vi "CommonVIs_OneButtonDialog.vi"(1 "message":string, 3 "yesButtonName":string="OK", 4 "noButtonName":string="Cancel", 5 "error in (no error)":errorcluster, 6 "WindowTitle":string, 7 "timeout(-1 ms) -1=infinity":i32=-1) -> (13 "timeOut":bool=TRUE, 16 "yesButtonPressed":bool, 19 "error out":errorcluster)   [LabVIEW 2014]
doc: "Displays a dialog box that contains a message and two buttons. <B>yesButtonName</B> and <B>noButtonName</B> are the names displayed on the buttons of the dialog box."
panel:
  in  "yesButton":bool
  out "showMessage":string
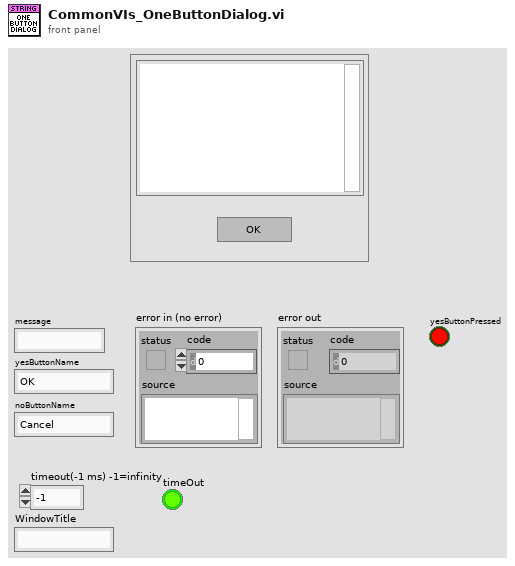
[diagram p1: front panel]
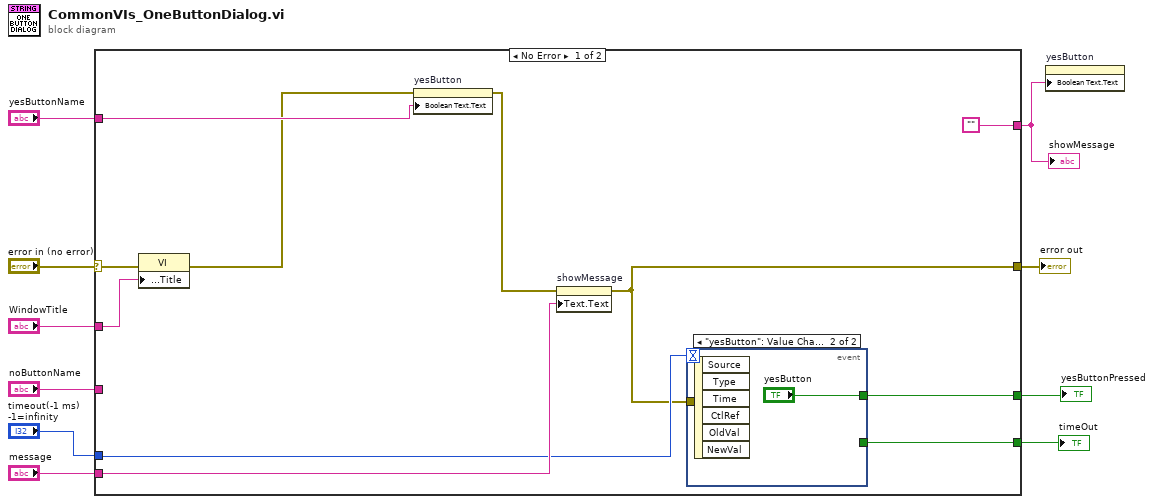
[diagram p0: block diagram]
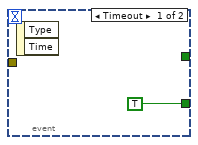
[diagram p2: hidden frame]
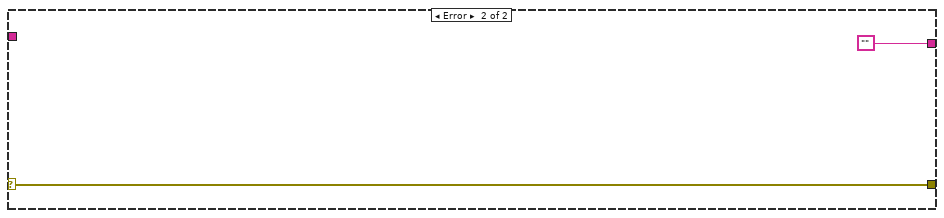
[diagram p3: hidden frame]
diagram:
  n1 = case shown="No Error" "error in (no error)" {
    selector: "error in (no error)" -> [w21 w25]
    tunnel: [w11 w25] -> w10
    tunnel: "noButtonName" -> [_ _]
    tunnel: "yesButtonName" -> [w19 _]
    tunnel: ["" ""] -> w6
    tunnel: "message" -> [w18 _]
    tunnel: "timeout(-1 ms) -1=infinity" -> [w17 _]
    tunnel: [w16 _] -> w3
    tunnel: [w15 _] -> w2
    tunnel: "WindowTitle" -> [w14 _]
    frame No Error {
      n2 = property class="VI"(error in=w21, "Front Panel Window:Title"=w14) -> (error out=w12:errorcluster)  [unwired: 1 in, 1 out]
      n3 = property on="yesButton" class="Bool"(error in=w12, "Boolean Text.Text"=w19) -> (error out=w13:errorcluster)  [unwired: 1 in, 1 out]
      n4 = property on="showMessage" class="Str"(error in=w13, "Text.Text"=w18) -> (error out=w11:errorcluster)  [unwired: 1 in, 1 out]
      n5 = event shown="[1] \"yesButton\": Value Change" {
        selector: _ -> [_ _]
        dyn-events: _ -> [_ _]
        timeout: w17 -> [_ _]
        tunnel: [TRUE _] -> w16
        tunnel: [_ "yesButton"] -> w15
        tunnel: w11 -> [_ _]
        event Timeout {
          n6 = event-data() -> ()  [unwired: 3 out]
        }
        event "yesButton": Value Change {
          n7 = event-data() -> ()  [unwired: 7 out]
        }
      }
    }
    frame Error {
    }
  }
  "error out" <- w10
  "yesButtonPressed" <- w2
  "showMessage" <- w6
  "timeOut" <- w3
  n8 = property on="yesButton" class="Bool"("Boolean Text.Text"=w6) -> ()  [unwired: 2 in, 2 out]
